vi "ScanAcquisitionDone.vi"(8 "error in (no error)":errorcluster, 11 "Camera_Controller_Comm in":refnum<class "Camera_Controller_Comm.lvclass">) -> (0 "error out":errorcluster, 3 "Camera_Controller_Comm out":refnum<class "Camera_Controller_Comm.lvclass">)   [LabVIEW 2023, in "Camera_Controller_Comm.lvlib" / "Camera_Controller_Comm.lvclass"]
uses:
  Camera_Controller_Comm.lvclass
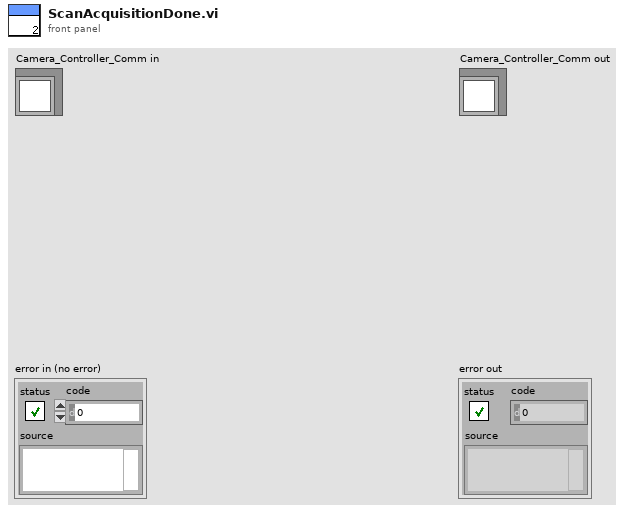
[diagram p1: front panel]
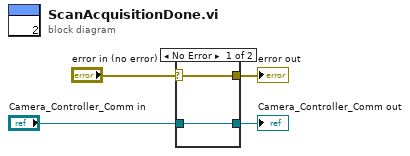
[diagram p0: block diagram]
diagram:
  n1 = case shown="No Error" "error in (no error)" {
    selector: "error in (no error)" -> [w5 w8]
    tunnel: [w5 w8] -> w3
    tunnel: [w6 w7] -> w1
    tunnel: "Camera_Controller_Comm in" -> [w6 w7]
    frame No Error {
    }
    frame Error {
    }
  }
  "error out" <- w3
  "Camera_Controller_Comm out" <- w1
